vi "conv.price.vi"(11 "price.in":sgl) -> (3 "price.out":u64 format="%.0x")   [LabVIEW 2020, in "fpganow.common.host.lvlib"]
uses:
  fpganow.common.host.lvlib
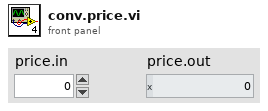
[diagram p1: front panel]
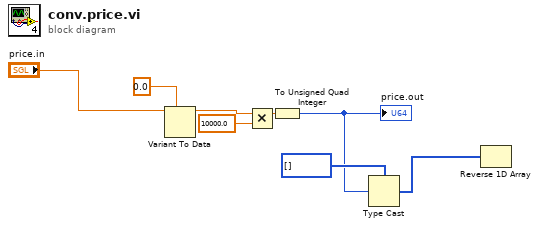
[diagram p0: block diagram]
diagram:
  n1 = Variant To Data(type=0.0, Variant="price.in") -> (data=w8:dbl)  [unwired: 1 in, 1 out]
  n2 = Multiply(x=w8, y=10000.0) -> (x*y=w4:dbl)
  n3 = To Unsigned Quad Integer(1:w4) -> (0:w1:u64)
  "price.out" <- w1
  n4 = Type Cast(type=u8[] [], x=w1) -> (*(type *) &x=w5:u8[])
  n5 = Reverse 1D Array(array=w5) -> ()  [unwired: 1 out]
